vi "initial.vi"(8 "error in (no error)":errorcluster, 11 "2410C-64 in":refnum<class "2410C-64.lvclass">) -> (0 "error out":errorcluster, 3 "2410C-64 out":refnum<class "2410C-64.lvclass">)   [LabVIEW 2019, in "2410C-64.lvclass"]
uses:
  2410C-64.lvclass
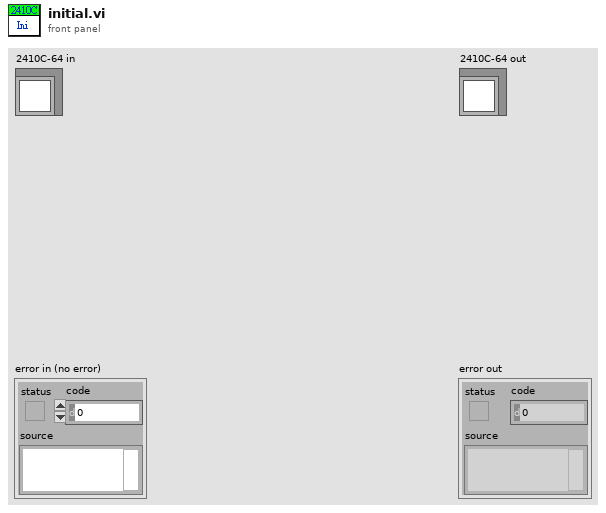
[diagram p1: front panel]
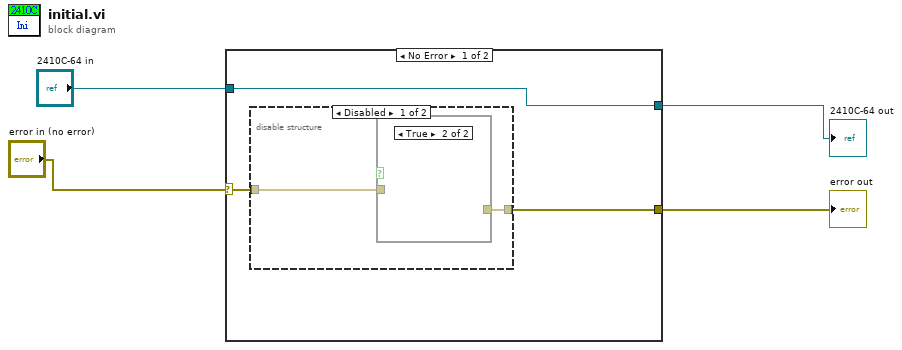
[diagram p0: block diagram]
diagram:
  n1 = case shown="No Error" "error in (no error)" {
    selector: "error in (no error)" -> [w6 w13]
    tunnel: [w7 w14] -> w3
    tunnel: "2410C-64 in" -> [w7 w14]
    tunnel: [w5 w13] -> w1
    frame No Error {
      n2 = disable-structure shown="Disabled" {
        disable-tunnel: w6 -> [w10 _]
        disable-tunnel: [w9 _] -> w5
        frame Disabled {
          n3 = case shown="True" w8 {
            tunnel: w10 -> [w11 _]
            tunnel: [w11 w12] -> w9
            frame False {
            }
            frame True {
            }
          }
        }
        frame Enabled {
        }
      }
    }
    frame Error {
    }
  }
  "error out" <- w1
  "2410C-64 out" <- w3
